vi "Starbuzz Coffee.vi"() -> ()   [LabVIEW 2013]
doc: "This is a test program to exercise the model for a coffee bistro sales application. It creates a few coffee drinks and embellishes them with various condiments. The final description and price of each drink is displayed to the user.\n\nThis example was redacted from the Java code provided in <i>Head First Design Patterns</i>, ISBN 0-596-00712-4"
uses:
  Classes/Espresso/Espresso.lvclass
  Classes/Dark Roast/Dark Roast.lvclass
  Classes/Milk/Milk.lvclass
  Classes/Mocha/Mocha.lvclass
  Classes/House Blend/House Blend.lvclass
  Classes/Soy/Soy.lvclass
  Classes/Whip/Whip.lvclass
  Classes/Abstract Beverage/Abstract Beverage.lvclass
  Classes/Condiment Decorator/Condiment Decorator.lvclass
panel:
  out "Your order":string
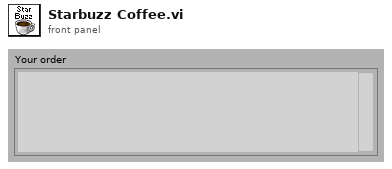
[diagram p1: front panel]
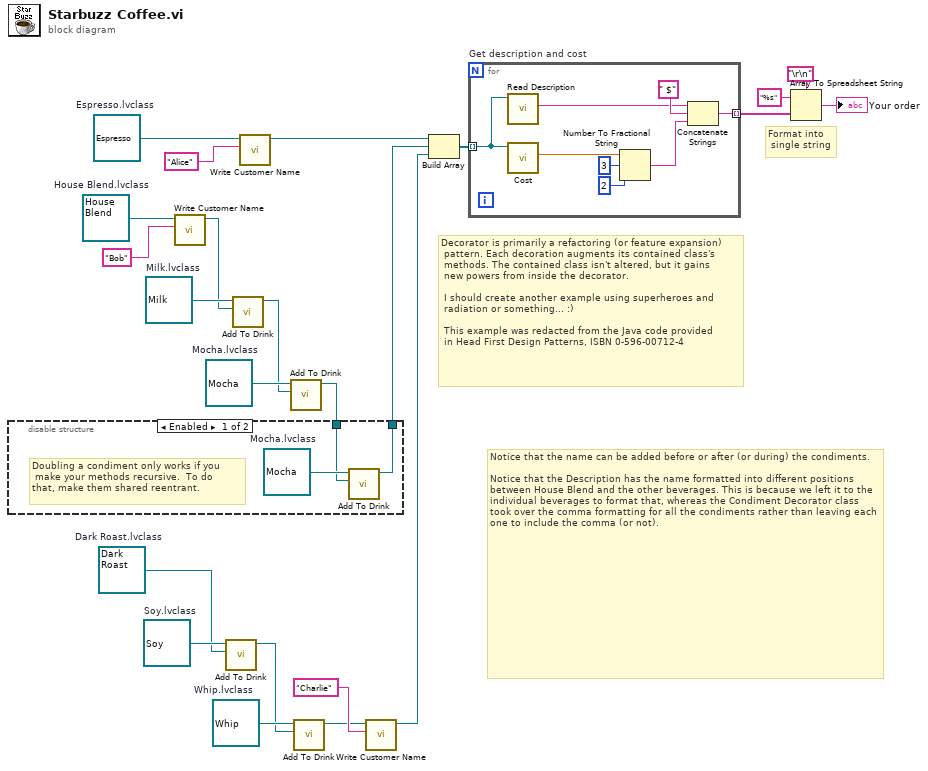
[diagram p0: block diagram]
diagram:
  w12 = refnum<class "Whip.lvclass"> refnum  # Whip.lvclass
  w13 = refnum<class "Soy.lvclass"> refnum  # Soy.lvclass
  w2 = refnum<class "House Blend.lvclass"> refnum  # House Blend.lvclass
  w22 = refnum<class "Mocha.lvclass"> refnum  # Mocha.lvclass
  w23 = refnum<class "Milk.lvclass"> refnum  # Milk.lvclass
  w1 = refnum<class "Dark Roast.lvclass"> refnum  # Dark Roast.lvclass
  w10 = refnum<class "Espresso.lvclass"> refnum  # Espresso.lvclass
  # "Notice that the name can be added before or after (or during) the condiments. \n\nNotice that the Description has the name formatted into different positions between House Blend and the other beverages. This is because we left it to the individual beverages to format that, whereas the Condiment Decorator class took over the comma formatting for all the condiments rather than leaving each one to include the comma (or not)."
  # "Format into\n single string"
  # "Decorator is primarily a refactoring (or feature expansion)\n pattern. Each decoration augments its contained class's \n methods. The contained class isn't altered, but it gains \n new powers from inside the decorator. \n\n I should create another example using superheroes and\n radiation or something... :)\n\n This example was redacted from the Java code provided\n in Head First Design Patterns, ISBN 0-596-00712-4"
  n1 = call-dynamic "Write Customer Name.vi"("Customer Name"="Bob", "Beverage in"=w2) -> ("Beverage in 2"=w6:refnum<class "House Blend.lvclass">)  [unwired: 9 in]
  n2 = call "Add To Drink.vi"("Abstract Beverage"=w1, "Condiment Decorator in"=w13) -> ("Condiment Decorator out"=w11:refnum<class "Soy.lvclass">)  [unwired: 9 in]
  n3 = call "Add To Drink.vi"("Abstract Beverage"=w6, "Condiment Decorator in"=w23) -> ("Condiment Decorator out"=w21:refnum<class "Milk.lvclass">)  [unwired: 9 in]
  n4 = call-dynamic "Write Customer Name.vi"("Customer Name"="Alice", "Beverage in"=w10) -> ("Beverage in 2"=w9:refnum<class "Espresso.lvclass">)  [unwired: 9 in]
  n5 = call "Add To Drink.vi"("Abstract Beverage"=w21, "Condiment Decorator in"=w22) -> ("Condiment Decorator out"=w20:refnum<class "Mocha.lvclass">)  [unwired: 9 in]
  n6 = disable-structure shown="Enabled" {
    disable-tunnel: w20 -> [w25 w27]
    disable-tunnel: [w24 w27] -> w19
    frame Enabled {
      w26 = refnum<class "Mocha.lvclass"> refnum  # Mocha.lvclass
      # "Doubling a condiment only works if you\n make your methods recursive.  To do\nthat, make them shared reentrant."
      n7 = call "Add To Drink.vi"("Abstract Beverage"=w25, "Condiment Decorator in"=w26) -> ("Condiment Decorator out"=w24:refnum<class "Mocha.lvclass">)  [unwired: 9 in]
    }
    frame Disabled {
    }
  }
  n8 = call "Add To Drink.vi"("Abstract Beverage"=w11, "Condiment Decorator in"=w12) -> ("Condiment Decorator out"=w4:refnum<class "Whip.lvclass">)  [unwired: 9 in]
  n9 = call-dynamic "Write Customer Name.vi"("Customer Name"="Charlie", "Condiment Decorator in"=w4) -> ("Condiment Decorator in 2"=w3:refnum<class "Whip.lvclass">)  [unwired: 9 in]
  n10 = Build Array(w9, w19, w3) -> (w18:refnum<class "Abstract Beverage.lvclass">[])
  n11 = for "Get description and cost" {
    tunnel: w18 -> [w28] mode=indexing
    tunnel: [w30] -> w16 mode=indexing
    n12 = call-dynamic "Read Description.vi"("Abstract Beverage in"=w28) -> ("Description"=w29:string)  [unwired: 10 in]
    n13 = call-dynamic "Cost.vi"("Abstract Beverage in"=w28) -> ("Cost"=w35:dbl)  [unwired: 8 in, 2 out]
    n14 = Number To Fractional String(number=w35, width (-)=i16 3, precision (6)=i16 2) -> (F-format string=w31:string)  [unwired: 1 in]
    n15 = Concatenate Strings(w29, " $" ("string"), w31) -> (w30:string)
  }
  n16 = Array To Spreadsheet String(delimiter (Tab)="\r\n", array=w16, 3:"%s" ("format string")) -> (spreadsheet string=→"Your order":string)
